vi "AAT2_FIR_FILTER_DESIGN_RECT_HAMMING.vi"() -> ()   [LabVIEW 2014]
uses:
  <vilib>/Analysis/NI_AALPro.lvlib
  <vilib>/measure/NI_MAPro.lvlib
panel:
  out "h'(n)":dbl[](array[numeric])
  out "Phase Response":dbl[](graph)
  out "Magnitude Response":dbl[](graph)
  in  "Graph Select":bool
  out "Filter Array hd(n)":dbl[](array[numeric])
  out "Window  Array":dbl[](array[numeric])
  in  "phase delay":dbl=350.0 format="%#.6g"
  in  "high cutoff freq: wu":dbl=350.0 format="%#.6g"
  in  "Filter Mode":T1(ring)
  in  "low cutoff freq: wc":dbl=150.0 format="%#.6g"
  in  "Window Mode":enum32{"Hamming", "Rectangular "}(ring)
  out "Time domain sketch":dbl[](graph)
  # "Window"
  # "Filter"
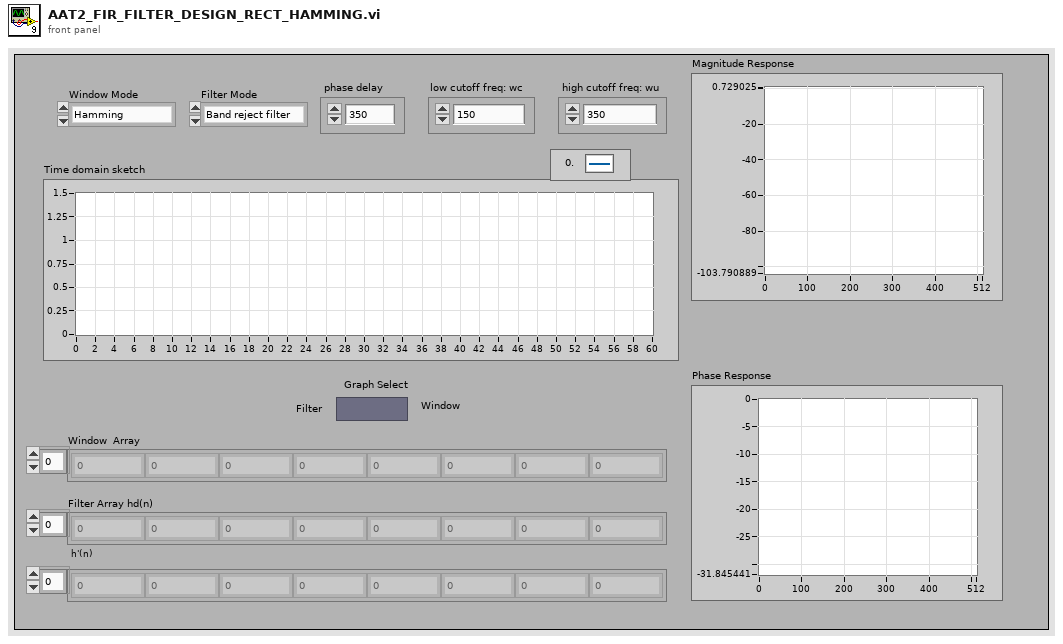
[diagram p1: front panel]
types:
  T1 = enum32{"Band reject filter", "band pass filter", "High pass filter", "Low pass filter"}
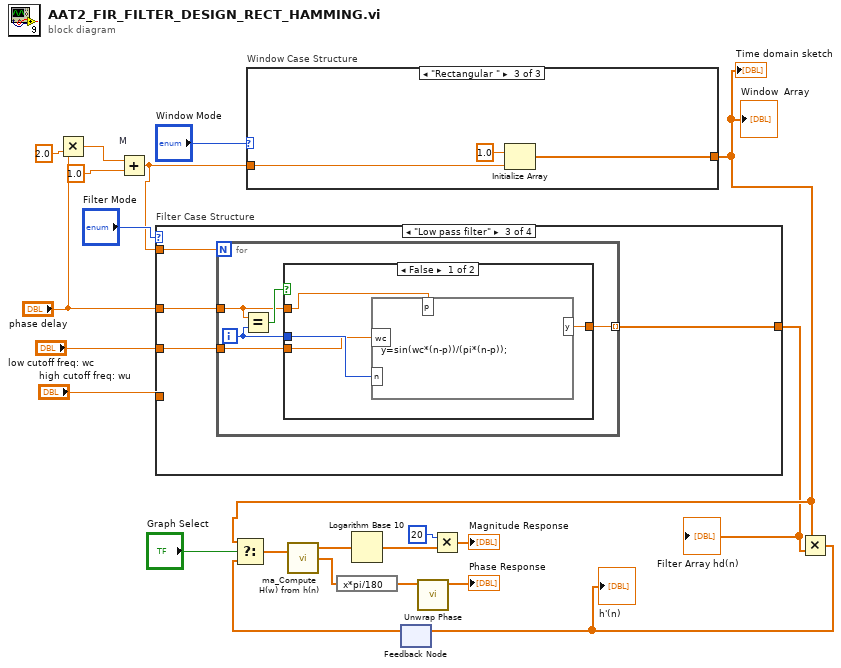
[diagram p0: block diagram]
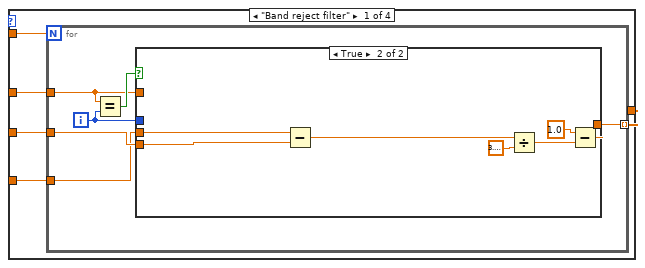
[diagram p2: hidden frame]
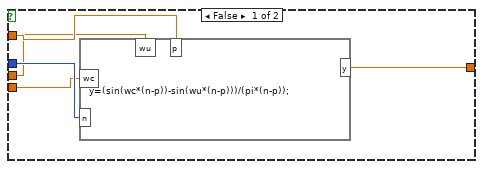
[diagram p3: hidden frame]
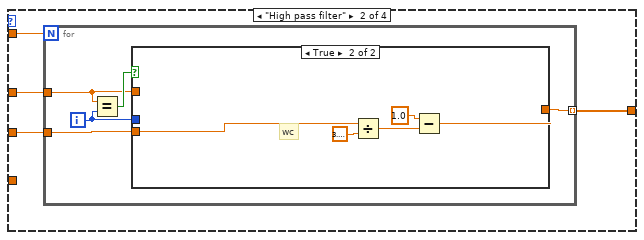
[diagram p4: hidden frame]
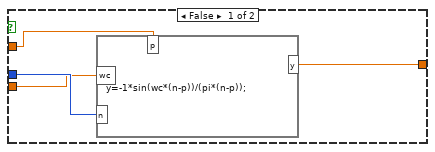
[diagram p5: hidden frame]
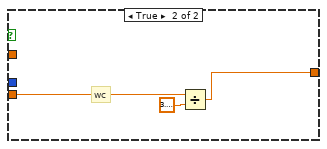
[diagram p6: hidden frame]
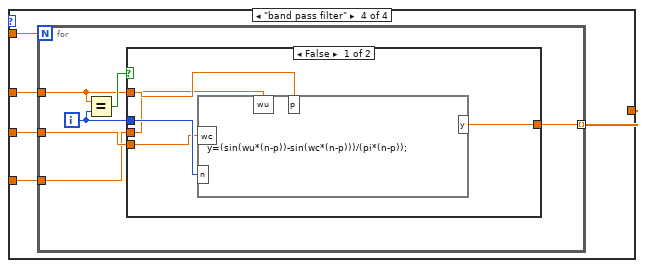
[diagram p7: hidden frame]
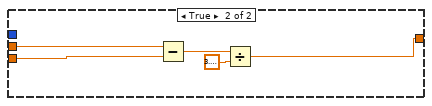
[diagram p8: hidden frame]
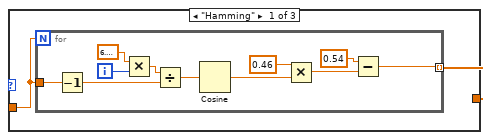
[diagram p9: hidden frame]
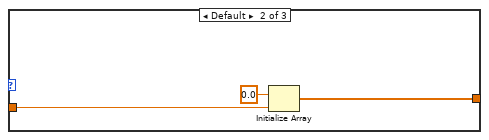
[diagram p10: hidden frame]
diagram:
  n1 = Multiply(x="phase delay", y=2.0) -> (x*y=w20:dbl)
  n2 = Add "M"(x=w20, y=1.0) -> (x+y=w4:dbl)
  n3 = case "Filter Case Structure" shown="\"Low pass filter\"" "Filter Mode" {
    tunnel: w4 -> [w27 w49 w67 w84]
    tunnel: "low cutoff freq: wc" -> [w24 w48 w66 w82]
    tunnel: "phase delay" -> [w26 w47 w65 w83]
    tunnel: [w23 w46 w64 w80] -> w3
    tunnel: "high cutoff freq: wu" -> [w25 _ _ w81]
    frame "Band reject filter" {
      n4 = for {
        N: w27 -> [_]
        tunnel: w26 -> [w30]
        tunnel: w24 -> [w32]
        tunnel: [w29] -> w23 mode=indexing
        tunnel: w25 -> [w28]
        i -> [w31]
        n5 = Equal?(x=w30, y=w31) -> (x = y?=w33:bool)
        n6 = case shown="True" w33 {
          tunnel: w32 -> [w37 w42]
          tunnel: w31 -> [w38 _]
          tunnel: w30 -> [w36 _]
          tunnel: [w35 w39] -> w29
          tunnel: w28 -> [w34 w43]
          frame False {
            n7 = formula code="y=(sin(wc*(n-p))-sin(wu*(n-p)))/(pi*(n-p));"("n"=w38, "wc"=w37, "p"=w36, "wu"=w34) -> ("y"=w35:dbl)
          }
          frame True {
            n8 = Subtract(x=w43, y=w42) -> (x-y=w44:dbl)
            n9 = Divide(x=w44, y=3.141592653589793) -> (x/y=w40:dbl)
            n10 = Subtract(x=1.0, y=w40) -> (x-y=w39:dbl)
          }
        }
      }
    }
    frame "High pass filter" {
      n11 = for {
        N: w49 -> [_]
        tunnel: w48 -> [w50]
        tunnel: w47 -> [w51]
        tunnel: [w52] -> w46 mode=indexing
        i -> [w53]
        n12 = Equal?(x=w51, y=w53) -> (x = y?=w54:bool)
        n13 = case shown="True" w54 {
          tunnel: w50 -> [w57 w59]
          tunnel: w53 -> [w58 _]
          tunnel: w51 -> [w56 _]
          tunnel: [w55 w60] -> w52
          frame False {
            n14 = formula code="y=-1*sin(wc*(n-p))/(pi*(n-p));"("n"=w58, "wc"=w57, "p"=w56) -> ("y"=w55:dbl)
          }
          frame True {
            # "wc"
            n15 = Divide(x=w59, y=3.141592653589793) -> (x/y=w61:dbl)
            n16 = Subtract(x=1.0, y=w61) -> (x-y=w60:dbl)
          }
        }
      }
    }
    frame "Low pass filter" {
      n17 = for {
        N: w67 -> [_]
        tunnel: w66 -> [w68]
        tunnel: w65 -> [w69]
        tunnel: [w70] -> w64 mode=indexing
        i -> [w71]
        n18 = Equal?(x=w69, y=w71) -> (x = y?=w72:bool)
        n19 = case shown="False" w72 {
          tunnel: w68 -> [w75 w78]
          tunnel: w71 -> [w76 _]
          tunnel: w69 -> [w74 _]
          tunnel: [w73 w77] -> w70
          frame False {
            n20 = formula code="y=sin(wc*(n-p))/(pi*(n-p));"("n"=w76, "wc"=w75, "p"=w74) -> ("y"=w73:dbl)
          }
          frame True {
            # "wc"
            n21 = Divide(x=w78, y=3.141592653589793) -> (x/y=w77:dbl)
          }
        }
      }
    }
    frame "band pass filter" {
      n22 = for {
        N: w84 -> [_]
        tunnel: w83 -> [w87]
        tunnel: w82 -> [w89]
        tunnel: [w86] -> w80 mode=indexing
        tunnel: w81 -> [w85]
        i -> [w88]
        n23 = Equal?(x=w87, y=w88) -> (x = y?=w90:bool)
        n24 = case shown="False" w90 {
          tunnel: w89 -> [w94 w96]
          tunnel: w88 -> [w95 _]
          tunnel: w87 -> [w93 _]
          tunnel: [w92 w98] -> w86
          tunnel: w85 -> [w91 w97]
          frame False {
            n25 = formula code="y=(sin(wu*(n-p))-sin(wc*(n-p)))/(pi*(n-p));"("n"=w95, "wc"=w94, "p"=w93, "wu"=w91) -> ("y"=w92:dbl)
          }
          frame True {
            n26 = Subtract(x=w97, y=w96) -> (x-y=w99:dbl)
            n27 = Divide(x=w99, y=3.141592653589793) -> (x/y=w98:dbl)
          }
        }
      }
    }
  }
  "Filter Array hd(n)" <- w3
  n28 = case "Window Case Structure" shown="\"Rectangular \"" "Window Mode" {
    tunnel: w4 -> [w101 w115 w118]
    tunnel: [w102 w114 w117] -> w5
    frame "Hamming" {
      # "This diagram executes if the Case Selector value is \"apple\"."
      n29 = for {
        N: w101 -> [_]
        tunnel: w101 -> [w108]
        tunnel: [w103] -> w102 mode=indexing
        i -> [w104]
        n30 = Decrement(x=w108) -> (x-1=w106:dbl)
        n31 = Multiply(x=6.283185307179586, y=w104) -> (x*y=w105:dbl)
        n32 = Divide(x=w105, y=w106) -> (x/y=w107:dbl)
        n33 = Cosine(x=w107) -> (cos(x)=w109:dbl)
        n34 = Multiply(x=0.46, y=w109) -> (x*y=w111:dbl)
        n35 = Subtract(x=0.54, y=w111) -> (x-y=w103:dbl)
      }
    }
    frame Default {
      n36 = Initialize Array(0.0 ("element"), w115) -> (w114:dbl[])
    }
    frame "Rectangular " {
      n37 = Initialize Array(1.0 ("element"), w118) -> (w117:dbl[])
    }
  }
  "Time domain sketch" <- w5
  "Window  Array" <- w5
  n38 = feedback #1() -> (w2:dbl[])  [unwired: 1 in]
  n39 = Select(t=w5, s="Graph Select", f=w2) -> (s? t:f=w10:dbl[])
  n40 = call <vilib>:"ma_Compute H(w) from h(n).vi"("h"=w10) -> ("Mag H(w)"=w12:dbl[], "Phase H(w)"=w14:dbl[])  [unwired: 1 in, 1 out]
  n41 = expression code="x*pi/180"(w14) -> (w13:dbl[])
  n42 = Logarithm Base 10(1:w12) -> (0:w7:dbl[])
  n43 = call <vilib>:"Unwrap Phase.vi"("Phase"=w13) -> ("Unwrapped Phase"=→"Phase Response":dbl[])  [unwired: 9 in, 1 out]
  n44 = Multiply(x=20, y=w7) -> (x*y=→"Magnitude Response":dbl[])
  n45 = Multiply(x=w5, y=w3) -> (x*y=w1:dbl[])
  "h'(n)" <- w1
  n46 = feedback-in #1(w1) -> ()
